vi "Initier attributs.vi"(8 "error in (no error)":errorcluster caption="entrée d'erreur (pas d'erreur)", 10 "Main/Refresh":string, 11 "UI SA en entrée":refnum<class "UI SmarAct.lvclass">) -> (0 "error out":errorcluster caption="sortie d'erreur", 3 "UI SA en sortie":refnum<class "UI SmarAct.lvclass">)   [LabVIEW 2024, in "UI SmarAct.lvclass"]
uses:
  UI SmarAct.lvclass
  Init Attributs.ctl
  UI SmarAct.lvclass/UI SmarAct.ctl
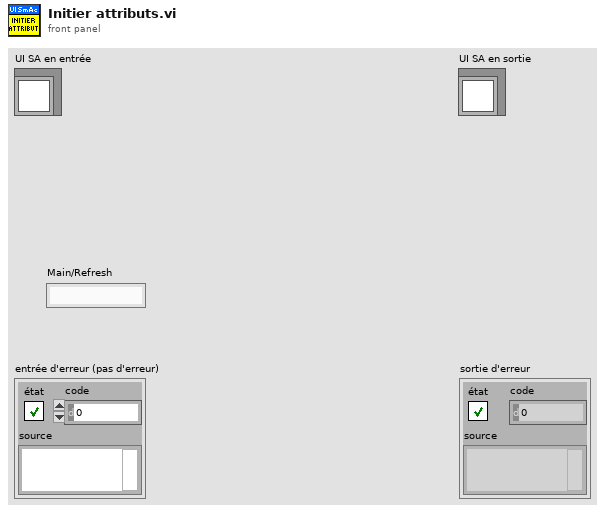
[diagram p1: front panel]
types:
  T1 = typedef "UI SmarAct.lvclass/Init Attributs.ctl" = enum16{"Init SelMCS", "InitConnect", "Init Connecter", "Init Channel", "Init Get Position", "Init Zero Position", "Init Find Zero", "Init Fréquence Max", "Init Vitesse Max", "Mode déplacement", "Init ctrl Spectro", "Init Tps Int-Cmde", "Init Spectre", "Switch Platine", "Init SMC 100", "Stop"}
  T2 = enum8{"Enabled", "Disabled", "Disabled and Grayed Out"}
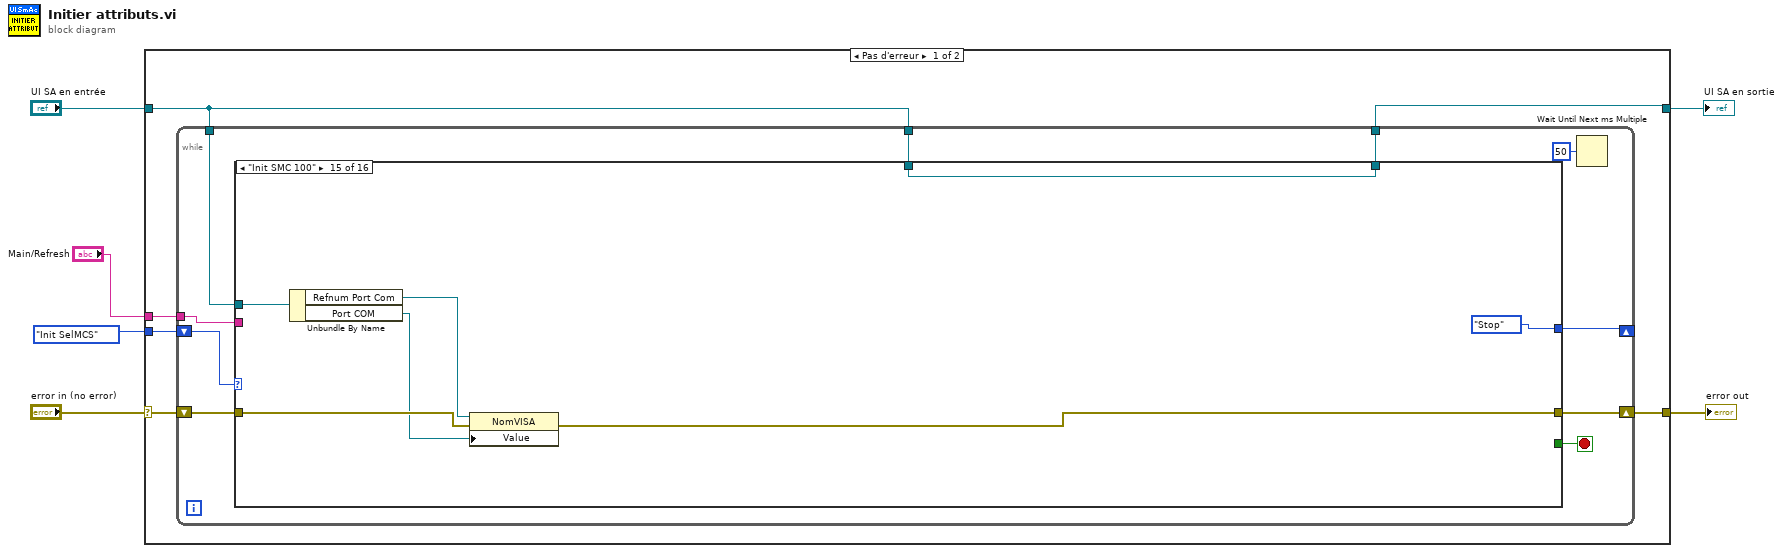
[diagram p0: block diagram]
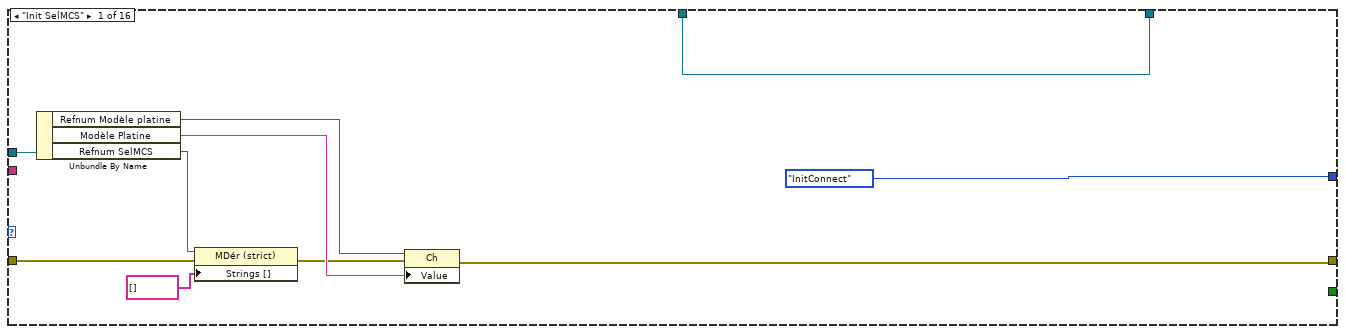
[diagram p2: hidden frame]
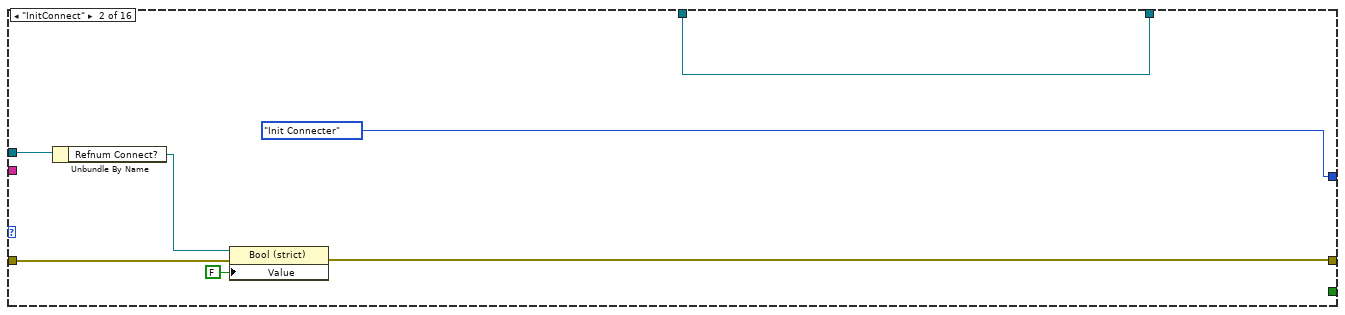
[diagram p3: hidden frame]
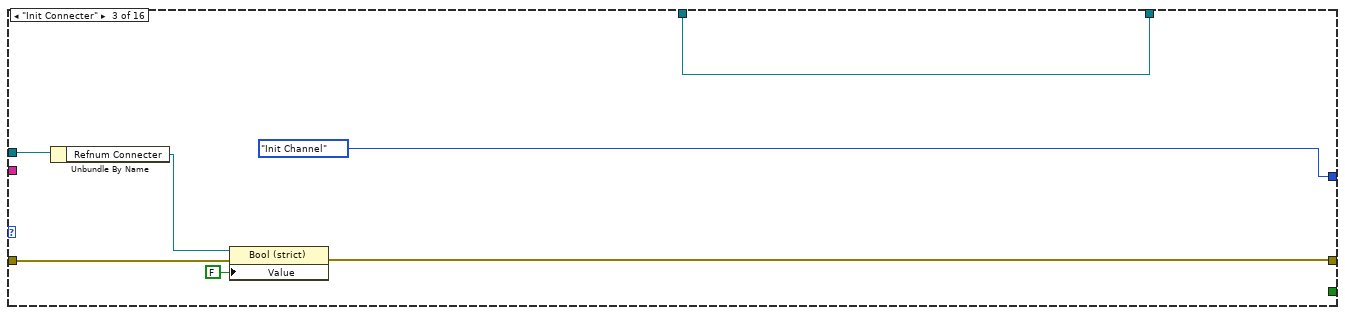
[diagram p4: hidden frame]
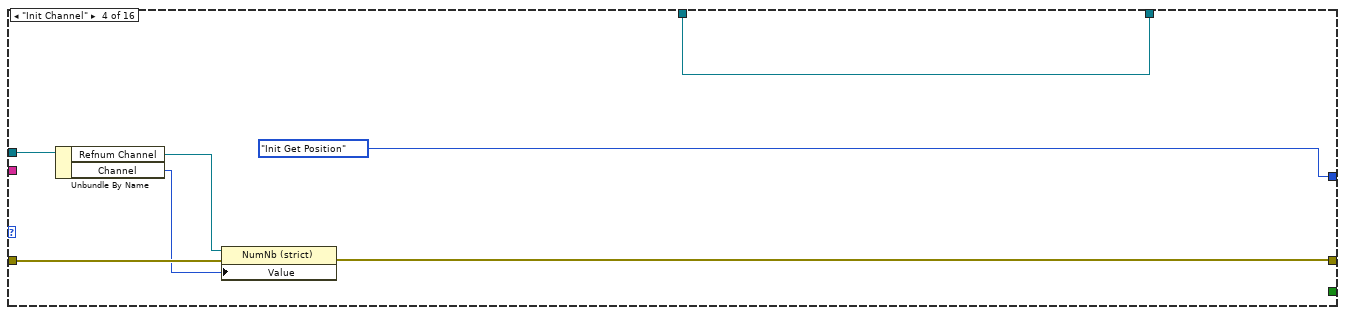
[diagram p5: hidden frame]
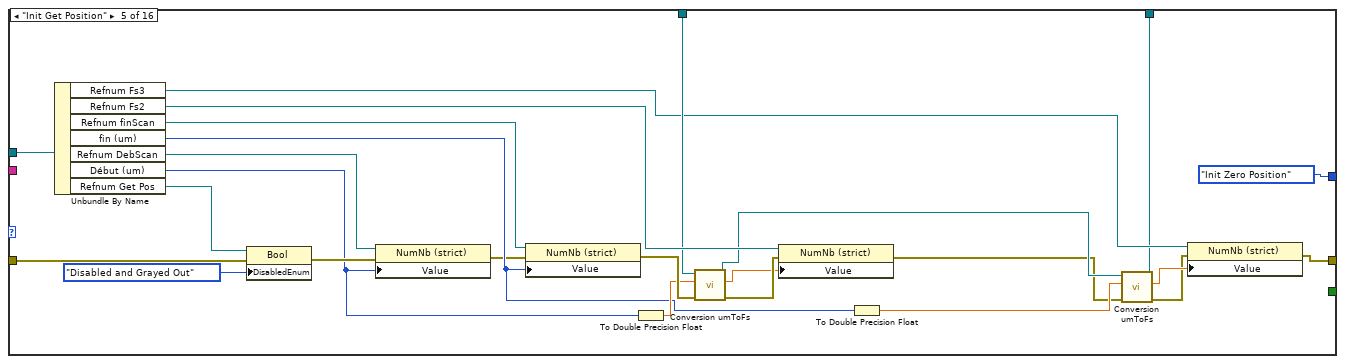
[diagram p6: hidden frame]
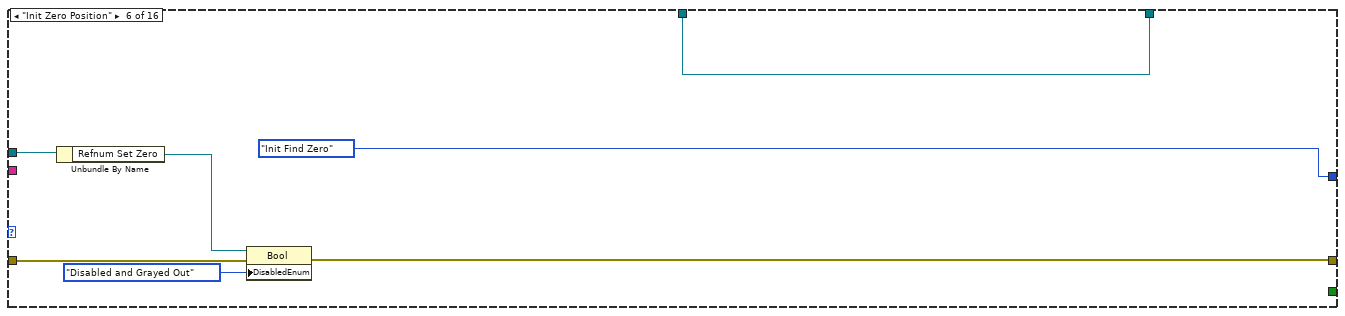
[diagram p7: hidden frame]
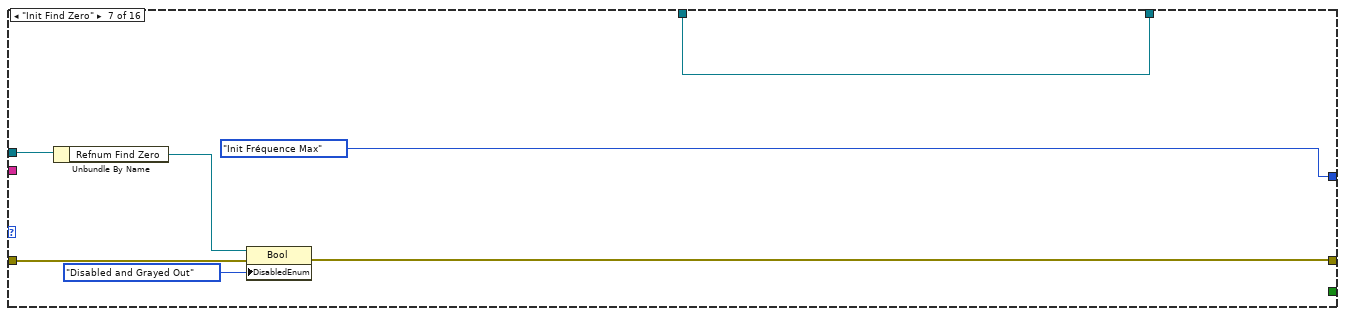
[diagram p8: hidden frame]
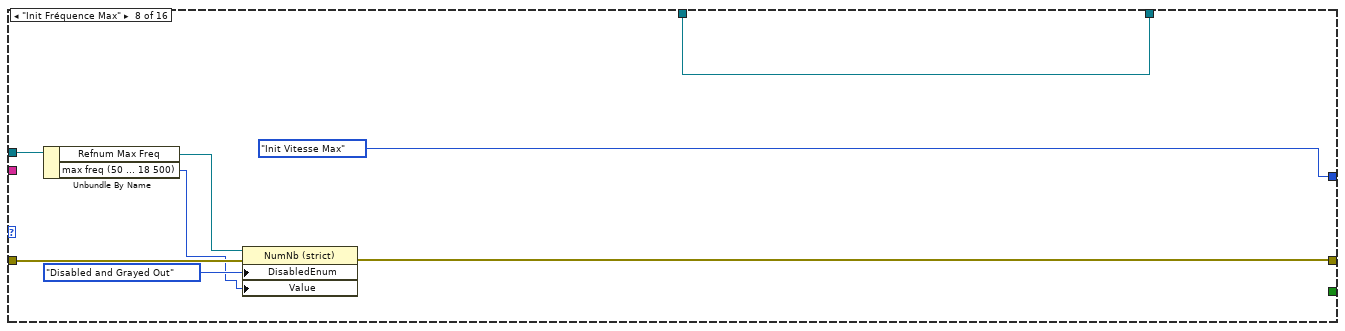
[diagram p9: hidden frame]
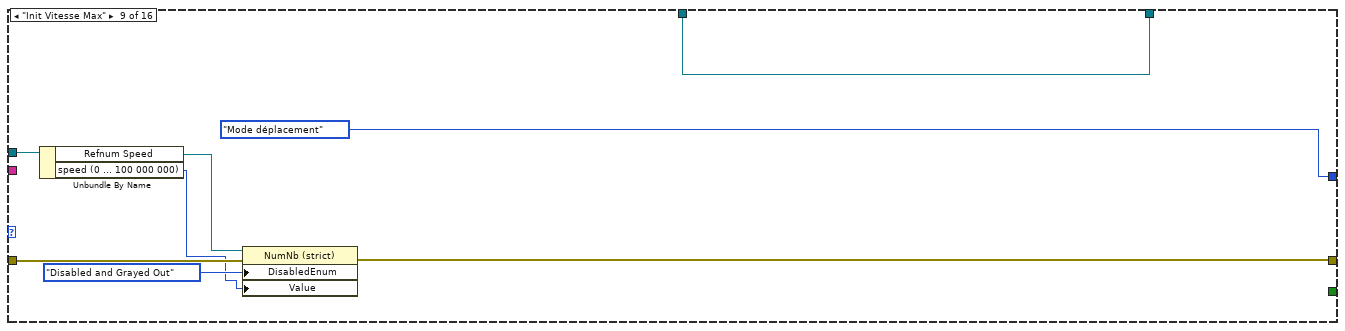
[diagram p10: hidden frame]
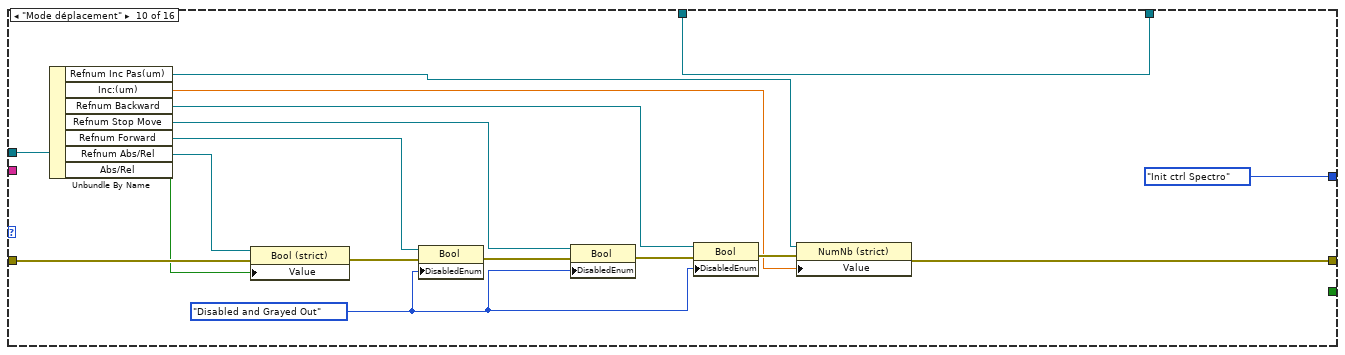
[diagram p11: hidden frame]
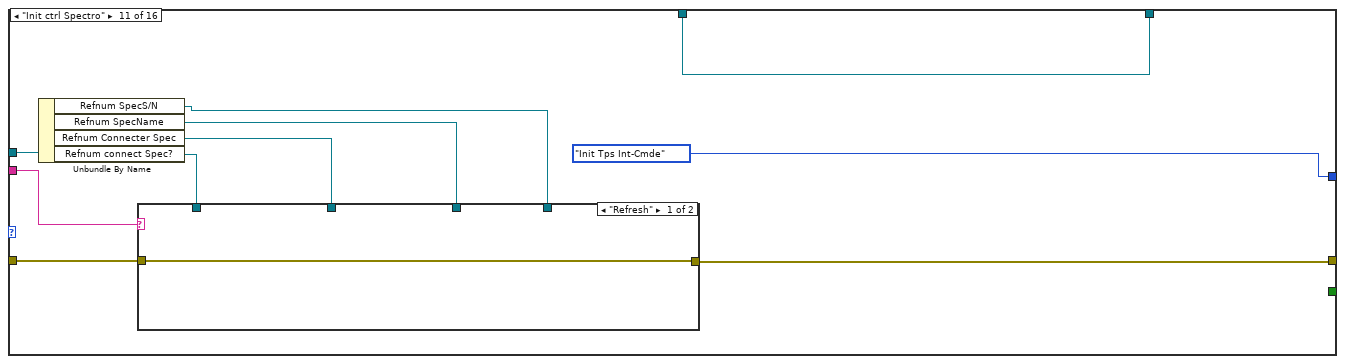
[diagram p12: hidden frame]
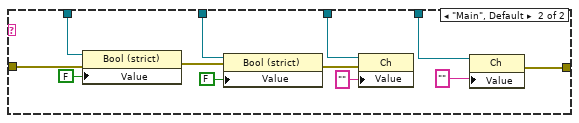
[diagram p13: hidden frame]
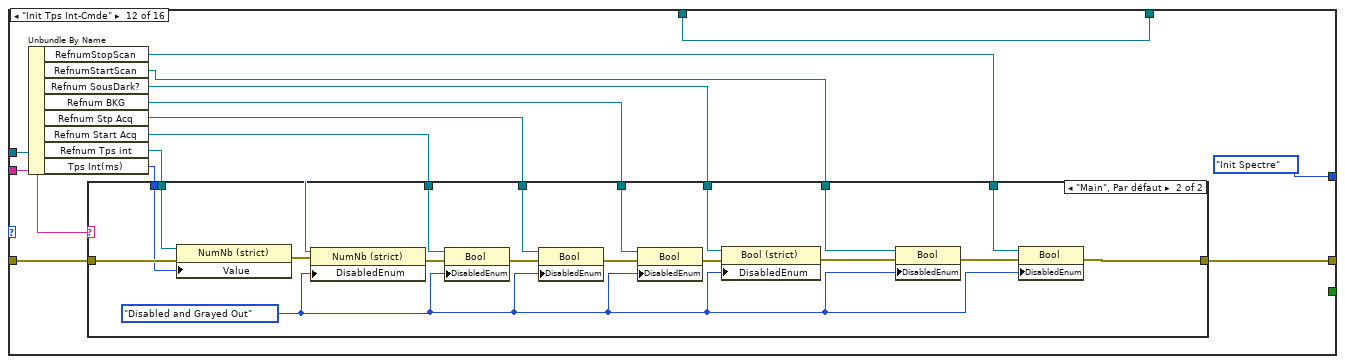
[diagram p14: hidden frame]
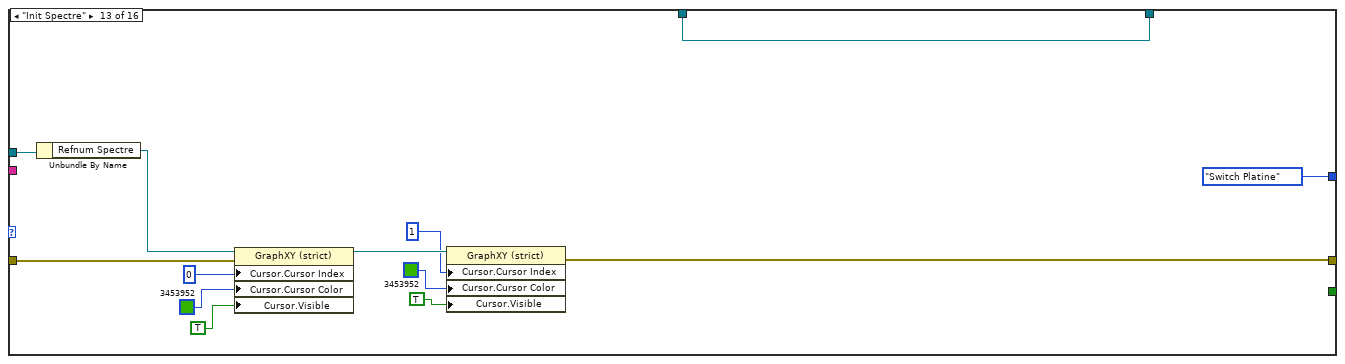
[diagram p16: hidden frame]
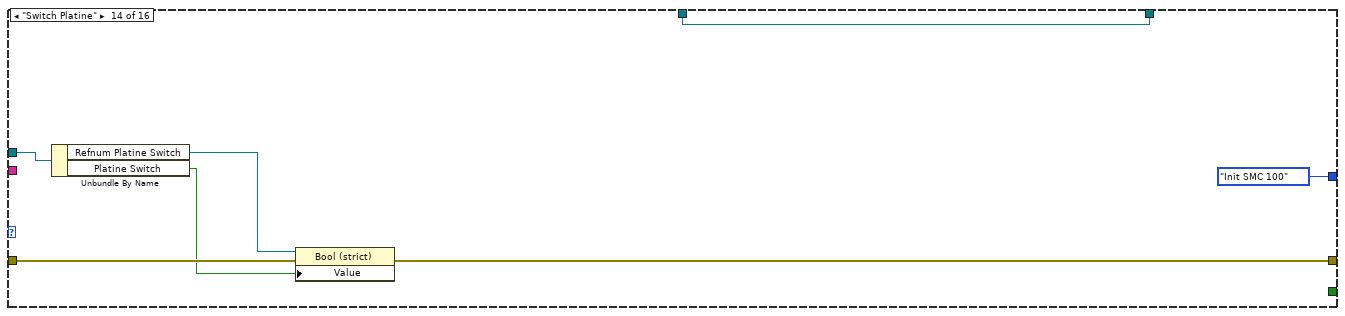
[diagram p17: hidden frame]
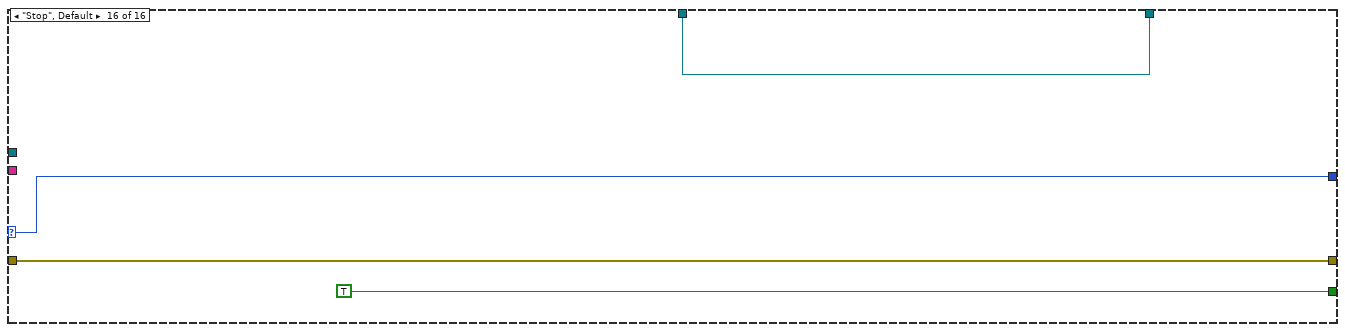
[diagram p18: hidden frame]
diagram:
  n1 = case shown="Pas d'erreur" "error in (no error)" {
    selector: "error in (no error)" -> [w12 w214]
    tunnel: [w11 w214] -> w5
    tunnel: [w7 w213] -> w3
    tunnel: "UI SA en entrée" -> [w8 w213]
    tunnel: Init_Attributs."Init SelMCS" -> [w10 _]
    tunnel: "Main/Refresh" -> [w9 _]
    frame No Error {
      n2 = while {
        shift-right: [w21] -> w11
        shift-left: w12 -> [w22]
        tunnel: w8 -> [w20]
        shift-right: [w18] -> _
        shift-left: w10 -> [w19]
        tunnel: w9 -> [w15]
        tunnel: w8 -> [w14]
        tunnel: [w13] -> w7
        stop <- w17 stop-if-true
        n3 = case shown="\"Init SMC 100\"" w19 {
          selector: w19 -> [_ _ _ _ _ _ _ _ _ _ _ _ _ _ _ w210]
          tunnel: w22 -> [w32 w38 w45 w52 w77 w84 w91 w99 w107 w124 w134 w161 w187 w198 w206 w212]
          tunnel: [w24 w37 w44 w51 w71 w83 w90 w98 w106 w111 w130 w157 w182 w197 w205 w212] -> w21
          tunnel: w20 -> [w30 w39 w46 w53 w78 w85 w92 w100 w108 w125 w135 w162 w194 w199 w204 _]
          tunnel: [Init_Attributs."InitConnect" Init_Attributs."Init Connecter" Init_Attributs."Init Channel" Init_Attributs."Init Get Position" Init_Attributs."Init Zero Position" Init_Attributs."Init Find Zero" Init_Attributs."Init Fréquence Max" Init_Attributs."Init Vitesse Max" Init_Attributs."Mode déplacement" Init_Attributs."Init ctrl Spectro" Init_Attributs."Init Tps Int-Cmde" Init_Attributs."Init Spectre" Init_Attributs."Switch Platine" Init_Attributs."Init SMC 100" Init_Attributs."Stop" w210] -> w18
          tunnel: [_ _ _ _ _ _ _ _ _ _ _ _ _ _ _ TRUE] -> w17
          tunnel: w15 -> [_ _ _ _ _ _ _ _ _ _ w127 w153 _ _ _ _]
          tunnel: w14 -> [w23 w33 w40 w47 w65 w79 w86 w93 w101 w113 w126 w151 w192 w201 w208 w209]
          tunnel: [w23 w33 w40 w47 w54 w79 w86 w93 w101 w113 w126 w151 w192 w201 w208 w209] -> w13
          frame "Init SelMCS" {
            n4 = Unbundle By Name(w30) -> ("Refnum Modèle platine"=w27:refnum<vi>, "Modèle Platine"=w26:string, "Refnum SelMCS"=w29:refnum<vi>)
            n5 = property class="MDér (strict)"(reference=w29, error in=w32, "Strings []"=string[] [] ("Chaînes []")) -> (error out=w25:errorcluster)  [unwired: 1 out]
            n6 = property class="Ch"(reference=w27, error in=w25, "Value"=w26) -> (error out=w24:errorcluster)  [unwired: 1 out]
          }
          frame "InitConnect" {
            n7 = Unbundle By Name(w39) -> ("Refnum Connect?"=w36:refnum<vi>)
            n8 = property class="Bool (strict)"(reference=w36, error in=w38, "Value"=FALSE ("Valeur")) -> (error out=w37:errorcluster)  [unwired: 1 out]
          }
          frame "Init Connecter" {
            n9 = Unbundle By Name(w46) -> ("Refnum Connecter"=w43:refnum<vi>)
            n10 = property class="Bool (strict)"(reference=w43, error in=w45, "Value"=FALSE ("Valeur")) -> (error out=w44:errorcluster)  [unwired: 1 out]
          }
          frame "Init Channel" {
            n11 = Unbundle By Name(w53) -> ("Refnum Channel"=w50:refnum<vi>, "Channel"=w48:u32)
            n12 = property class="NumNb (strict)"(reference=w50, error in=w52, "Value"=w48) -> (error out=w51:errorcluster)  [unwired: 1 out]
          }
          frame "Init Get Position" {
            n13 = Unbundle By Name(w78) -> ("Refnum Fs3"=w58:refnum<vi>, "Refnum Fs2"=w69:refnum<vi>, "Refnum finScan"=w70:refnum<vi>, "fin (um)"=w62:i32, "Refnum DebScan"=w73:refnum<vi>, "Début (um)"=w64:i32, "Refnum Get Pos"=w76:refnum<vi>)
            n14 = property class="Bool"(reference=w76, error in=w77, "DisabledEnum"=T2."Disabled and Grayed Out" ("Désactivée")) -> (error out=w72:errorcluster)  [unwired: 1 out]
            n15 = property class="NumNb (strict)"(reference=w73, error in=w72, "Value"=w64) -> (error out=w55:errorcluster)  [unwired: 1 out]
            n16 = property class="NumNb (strict)"(reference=w70, error in=w55, "Value"=w62) -> (error out=w68:errorcluster)  [unwired: 1 out]
            n17 = To Double Precision Float(number=w64) -> (double precision float=w63:dbl)
            n18 = call "Conversion umToFs.vi"("error in (no error)"=w68, "um"=w63, "UI SA en entrée"=w65) -> ("error out"=w67:errorcluster, "Fs"=w66:ext, "UI SA en sortie"=w60:refnum<class "UI SmarAct.lvclass">)  [unwired: 6 in]
            n19 = property class="NumNb (strict)"(reference=w69, error in=w67, "Value"=w66) -> (error out=w59:errorcluster)  [unwired: 1 out]
            n20 = To Double Precision Float(number=w62) -> (double precision float=w61:dbl)
            n21 = call "Conversion umToFs.vi"("error in (no error)"=w59, "um"=w61, "UI SA en entrée"=w60) -> ("error out"=w56:errorcluster, "Fs"=w57:ext, "UI SA en sortie"=w54:refnum<class "UI SmarAct.lvclass">)  [unwired: 6 in]
            n22 = property class="NumNb (strict)"(reference=w58, error in=w56, "Value"=w57) -> (error out=w71:errorcluster)  [unwired: 1 out]
          }
          frame "Init Zero Position" {
            n23 = Unbundle By Name(w85) -> ("Refnum Set Zero"=w82:refnum<vi>)
            n24 = property class="Bool"(reference=w82, error in=w84, "DisabledEnum"=T2."Disabled and Grayed Out" ("Désactivée")) -> (error out=w83:errorcluster)  [unwired: 1 out]
          }
          frame "Init Find Zero" {
            n25 = Unbundle By Name(w92) -> ("Refnum Find Zero"=w89:refnum<vi>)
            n26 = property class="Bool"(reference=w89, error in=w91, "DisabledEnum"=T2."Disabled and Grayed Out" ("Désactivée")) -> (error out=w90:errorcluster)  [unwired: 1 out]
          }
          frame "Init Fréquence Max" {
            n27 = Unbundle By Name(w100) -> ("Refnum Max Freq"=w97:refnum<vi>, "max freq (50 ... 18 500)"=w94:u32)
            n28 = property class="NumNb (strict)"(reference=w97, error in=w99, "DisabledEnum"=T2."Disabled and Grayed Out" ("Désactivée"), "Value"=w94) -> (error out=w98:errorcluster)  [unwired: 1 out]
          }
          frame "Init Vitesse Max" {
            n29 = Unbundle By Name(w108) -> ("Refnum Speed"=w105:refnum<vi>, "speed (0 ... 100 000 000)"=w102:u32)
            n30 = property class="NumNb (strict)"(reference=w105, error in=w107, "DisabledEnum"=T2."Disabled and Grayed Out" ("Désactivée"), "Value"=w102) -> (error out=w106:errorcluster)  [unwired: 1 out]
          }
          frame "Mode déplacement" {
            w114 = T2."Disabled and Grayed Out" ("Désactivée")
            n31 = Unbundle By Name(w125) -> ("Refnum Inc Pas(um)"=w110:refnum<vi>, "Inc:(um)"=w109:dbl, "Refnum Backward"=w118:refnum<vi>, "Refnum Stop Move"=w119:refnum<vi>, "Refnum Forward"=w120:refnum<vi>, "Refnum Abs/Rel"=w123:refnum<vi>, "Abs/Rel"=w121:bool)
            n32 = property class="Bool (strict)"(reference=w123, error in=w124, "Value"=w121) -> (error out=w115:errorcluster)  [unwired: 1 out]
            n33 = property class="Bool"(reference=w120, error in=w115, "DisabledEnum"=w114) -> (error out=w116:errorcluster)  [unwired: 1 out]
            n34 = property class="Bool"(reference=w119, error in=w116, "DisabledEnum"=w114) -> (error out=w117:errorcluster)  [unwired: 1 out]
            n35 = property class="Bool"(reference=w118, error in=w117, "DisabledEnum"=w114) -> (error out=w112:errorcluster)  [unwired: 1 out]
            n36 = property class="NumNb (strict)"(reference=w110, error in=w112, "Value"=w109) -> (error out=w111:errorcluster)  [unwired: 1 out]
          }
          frame "Init ctrl Spectro" {
            n37 = Unbundle By Name(w135) -> ("Refnum SpecS/N"=w128:refnum<vi>, "Refnum SpecName"=w129:refnum<vi>, "Refnum Connecter Spec"=w131:refnum<vi>, "Refnum connect Spec?"=w133:refnum<vi>)
            n38 = case shown="\"Refresh\"" w127 {
              tunnel: w134 -> [w136 w148]
              tunnel: w133 -> [_ w147]
              tunnel: w131 -> [_ w144]
              tunnel: [w136 w141] -> w130
              tunnel: w129 -> [_ w140]
              tunnel: w128 -> [_ w139]
              frame "Refresh" {
              }
              frame "Main", Default {
                n39 = property class="Bool (strict)"(reference=w147, error in=w148, "Value"=FALSE ("Valeur")) -> (error out=w145:errorcluster)  [unwired: 1 out]
                n40 = property class="Bool (strict)"(reference=w144, error in=w145, "Value"=FALSE ("Valeur")) -> (error out=w142:errorcluster)  [unwired: 1 out]
                n41 = property class="Ch"(reference=w140, error in=w142, "Value"="" ("Valeur")) -> ()  [unwired: 2 out]
                n42 = property class="Ch"(reference=w139, "Value"="" ("Valeur")) -> (error out=w141:errorcluster)  [unwired: 1 in, 1 out]
              }
            }
          }
          frame "Init Tps Int-Cmde" {
            n43 = Unbundle By Name(w162) -> ("RefnumStopScan"=w149:refnum<vi>, "RefnumStartScan"=w150:refnum<vi>, "Refnum SousDark?"=w152:refnum<vi>, "Refnum BKG"=w154:refnum<vi>, "Refnum Stp Acq"=w155:refnum<vi>, "Refnum Start Acq"=w156:refnum<vi>, "Refnum Tps int"=w158:refnum<vi>, "Tps Int(ms)"=w159:u32)
            n44 = case shown="\"Main\", Par défaut" w153 {
              tunnel: w161 -> [w163 w181]
              tunnel: w159 -> [_ w179]
              tunnel: w158 -> [_ w178]
              tunnel: [w163 w168] -> w157
              tunnel: w156 -> [_ w174]
              tunnel: w155 -> [_ w173]
              tunnel: w154 -> [_ w172]
              tunnel: w152 -> [_ w170]
              tunnel: w150 -> [_ w166]
              tunnel: w149 -> [_ w165]
              frame "Refresh" {
              }
              frame "Main", Default {
                w164 = T2."Disabled and Grayed Out" ("Désactivée")
                n45 = property class="NumNb (strict)"(reference=w178, error in=w181, "Value"=w179) -> (error out=w180:errorcluster)  [unwired: 1 out]
                n46 = property class="NumNb (strict)"(reference=w178, error in=w180, "DisabledEnum"=w164) -> (error out=w177:errorcluster)  [unwired: 1 out]
                n47 = property class="Bool"(reference=w174, error in=w177, "DisabledEnum"=w164) -> (error out=w176:errorcluster)  [unwired: 1 out]
                n48 = property class="Bool"(reference=w173, error in=w176, "DisabledEnum"=w164) -> (error out=w175:errorcluster)  [unwired: 1 out]
                n49 = property class="Bool"(reference=w172, error in=w175, "DisabledEnum"=w164) -> (error out=w171:errorcluster)  [unwired: 1 out]
                n50 = property class="Bool (strict)"(reference=w170, error in=w171, "DisabledEnum"=w164) -> (error out=w167:errorcluster)  [unwired: 1 out]
                n51 = property class="Bool"(reference=w166, error in=w167, "DisabledEnum"=w164) -> (error out=w169:errorcluster)  [unwired: 1 out]
                n52 = property class="Bool"(reference=w165, error in=w169, "DisabledEnum"=w164) -> (error out=w168:errorcluster)  [unwired: 1 out]
              }
            }
          }
          frame "Init Spectre" {
            n53 = Unbundle By Name(w194) -> ("Refnum Spectre"=w191:refnum<vi>)
            n54 = property class="GraphXY (strict)"(reference=w191, error in=w187, "Cursor.Cursor Index"=0 ("Curseur.Indice du curseur"), "Cursor.Cursor Color"=u32 3453952, "Cursor.Visible"=TRUE ("Curseur.Visible")) -> (reference out=w186:refnum<vi>)  [unwired: 1 out]
            n55 = property class="GraphXY (strict)"(reference=w186, "Cursor.Cursor Index"=1 ("Curseur.Indice du curseur"), "Cursor.Cursor Color"=u32 3453952, "Cursor.Visible"=TRUE ("Curseur.Visible")) -> (error out=w182:errorcluster)  [unwired: 1 in, 1 out]
          }
          frame "Switch Platine" {
            n56 = Unbundle By Name(w199) -> ("Refnum Platine Switch"=w196:refnum<vi>, "Platine Switch"=w195:bool)
            n57 = property class="Bool (strict)"(reference=w196, error in=w198, "Value"=w195) -> (error out=w197:errorcluster)  [unwired: 1 out]
          }
          frame "Init SMC 100" {
            n58 = Unbundle By Name(w204) -> ("Refnum Port Com"=w203:refnum<vi>, "Port COM"=w202:refnum<visa-resource-name>)
            n59 = property class="NomVISA"(reference=w203, error in=w206, "Value"=w202) -> (error out=w205:errorcluster)  [unwired: 1 out]
          }
          frame "Stop", Default {
          }
        }
        n60 = Wait Until Next ms Multiple(millisecond multiple=u32 50 ("n millisecondes")) -> ()  [unwired: 1 out]
      }
    }
    frame Error {
    }
  }
  "error out" <- w5
  "UI SA en sortie" <- w3
